vi "Intensity Graph Linecut (Vertical) (by val).vi"(6 "Averaging Method":enum16{"Step", "Gaussian"}(ring), 8 "error in (no error)":errorcluster, 9 "width (vertical)":dbl, 10 "2D Data":dbl[][](array[numeric]), 11 "graph_utilities in":refnum<class "graph_utilities.lvclass">) -> (0 "error out":errorcluster, 2 "XY-data":cluster{"X-array":dbl[], "Y-array":dbl[]}[](array[cluster]), 3 "graph_utilities out":refnum<class "graph_utilities.lvclass">)   [LabVIEW 2019, in "graph_utilities.lvclass"]
doc: "Takes a Vertical Linecut of an Intensity Graph and outputs to an XY Graph. The center location of the linecut is determined by the x-position of the Intensity Graph's curser.\n - <b>width</b> is the standard deviation of a Gaussian function in the units of the Intensity Graph x scale.\n - If <b>width = 0 </b> the spacing between two adjacent data points will be used."
uses:
  graph_utilities.lvclass
  <vilib>/Analysis/NI_AALBase.lvlib
  <vilib>/Analysis/baseanly.llb/A x Vector.vi
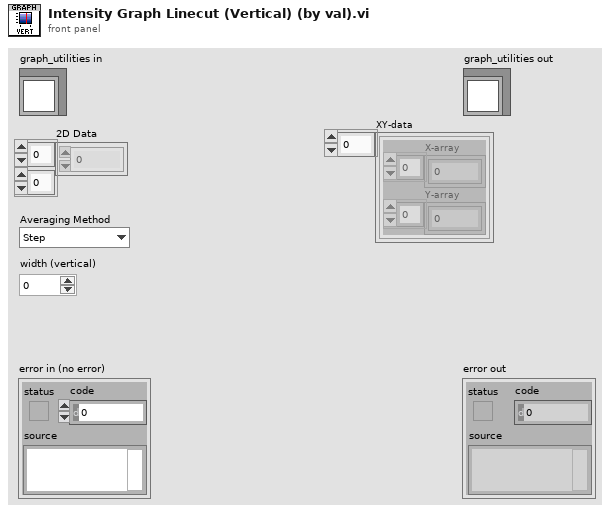
[diagram p1: front panel]
types:
  T1 = typedef "LVPointDoubleTypeDef.ctl" = cluster{"X":dbl, "Y":dbl}
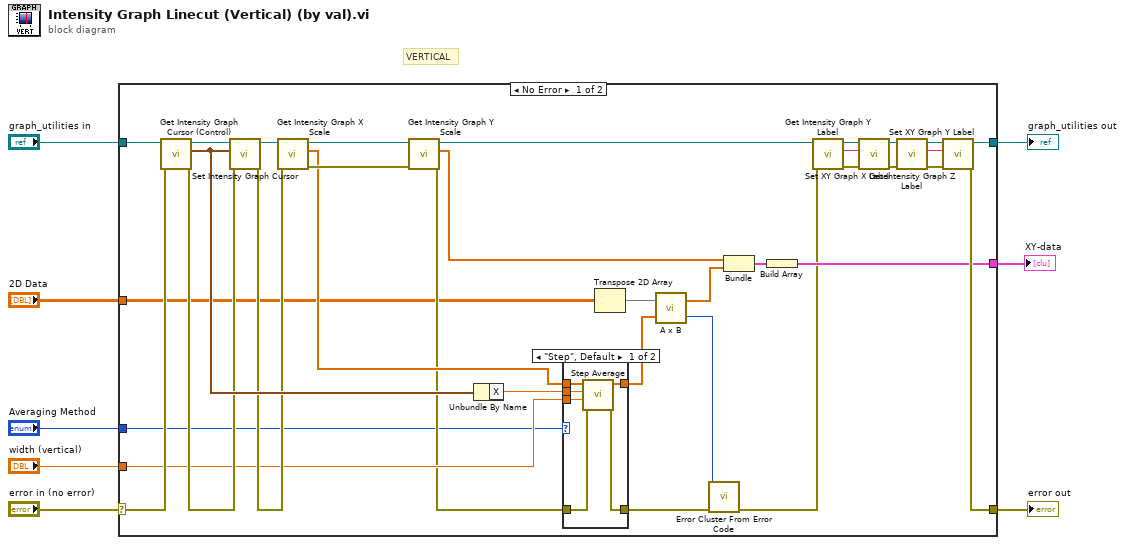
[diagram p0: block diagram]
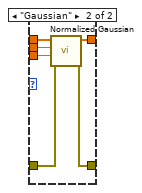
[diagram p2: hidden frame]
diagram:
  # "VERTICAL"
  n1 = case shown="No Error" "error in (no error)" {
    selector: "error in (no error)" -> [w36 w57]
    tunnel: [w14 w57] -> w7
    tunnel: [w13 w56] -> w5
    tunnel: "graph_utilities in" -> [w39 w56]
    tunnel: "width (vertical)" -> [w28 _]
    tunnel: "Averaging Method" -> [w12 _]
    tunnel: "2D Data" -> [w11 _]
    tunnel: [w10 _] -> w1
    frame No Error {
      n2 = call "Get Intensity Graph Cursor (Control).vi"("error in (no error)"=w36, "graph_utilities in"=w39) -> ("error out"=w35:errorcluster, "Cursor.Cursor Position"=w37:T1, "graph_utilities out"=w40:refnum<class "graph_utilities.lvclass">)  [unwired: 7 in]
      n3 = call "Set Intensity Graph Cursor.vi"("error in (no error)"=w35, "Cursor.Cursor Position"=w37, "graph_utilities in"=w40) -> ("error out"=w34:errorcluster, "graph_utilities out"=w38:refnum<class "graph_utilities.lvclass">)  [unwired: 7 in]
      n4 = call "Get Intensity Graph X Scale.vi"("error in (no error)"=w34, "graph_utilities in"=w38) -> ("error out"=w32:errorcluster, "X Scale"=w30:dbl[], "graph_utilities out"=w33:refnum<class "graph_utilities.lvclass">)  [unwired: 6 in, 1 out]
      n5 = call "Get Intensity Graph Y Scale.vi"("error in (no error)"=w32, "graph_utilities in"=w33) -> ("error out"=w26:errorcluster, "Y Scale"=w31:dbl[], "graph_utilities out"=w23:refnum<class "graph_utilities.lvclass">)  [unwired: 6 in, 1 out]
      n6 = Unbundle By Name(w37) -> ("X"=w29:dbl)
      n7 = case shown="\"Step\", Default" w12 {
        tunnel: w30 -> [w49 w55]
        tunnel: w29 -> [w48 w54]
        tunnel: w28 -> [w47 w53]
        tunnel: [w45 w52] -> w27
        tunnel: w26 -> [w46 w51]
        tunnel: [w44 w50] -> w25
        frame "Step", Default {
          n8 = call "Step Average.vi"("error in (no error)"=w46, "width (c)"=w47, "position (b)"=w48, "Scale"=w49) -> ("error out"=w44:errorcluster, "Averaged Result"=w45:dbl[])  [unwired: 4 in, 2 out]
        }
        frame "Gaussian" {
          n9 = call "Normalized Gaussian.vi"("error in (no error)"=w51, "width (c)"=w53, "position (b)"=w54, "Scale"=w55) -> ("error out"=w50:errorcluster, "Normalized Gaussian"=w52:dbl[])  [unwired: 6 in]
        }
      }
      n10 = Transpose 2D Array(2D array=w11) -> (transposed array=w43:dbl[][])
      n11 = call-poly <vilib>:"A x B.vi"("Vector"=w27, "A"=w43) -> ("error"=w41:i32, "A x Vector"=w42:dbl[])
      n12 = call <vilib>:"Error Cluster From Error Code.vi"("error in (no error)"=w25, "error code (0)"=w41) -> ("error out"=w9:errorcluster)  [unwired: 7 in]
      n13 = Bundle("Y Scale"=w31, "A x Vector"=w42) -> (w24:cluster{"Y Scale":dbl[], "A x Vector":dbl[]})  [unwired: 1 in]
      n14 = Build Array(w24) -> (w10:cluster{"Y Scale":dbl[], "A x Vector":dbl[]}[])
      n15 = call "Get Intensity Graph Y Label.vi"("error in (no error)"=w9, "graph_utilities in"=w23) -> ("error out"=w17:errorcluster, "Y Label"=w19:string, "graph_utilities out"=w18:refnum<class "graph_utilities.lvclass">)  [unwired: 7 in]
      n16 = call "Set XY Graph X Label.vi"("error in (no error)"=w17, "X Label"=w19, "graph_utilities in"=w18) -> ("error out"=w15:errorcluster, "graph_utilities out"=w16:refnum<class "graph_utilities.lvclass">)  [unwired: 7 in]
      n17 = call "Get Intensity Graph Z Label.vi"("error in (no error)"=w15, "graph_utilities in"=w16) -> ("error out"=w20:errorcluster, "Z Label"=w22:string, "graph_utilities out"=w21:refnum<class "graph_utilities.lvclass">)  [unwired: 7 in]
      n18 = call "Set XY Graph Y Label.vi"("error in (no error)"=w20, "Y Label"=w22, "graph_utilities in"=w21) -> ("error out"=w14:errorcluster, "graph_utilities out"=w13:refnum<class "graph_utilities.lvclass">)  [unwired: 7 in]
    }
    frame Error {
    }
  }
  "error out" <- w7
  "graph_utilities out" <- w5
  "XY-data" <- w1
